vi "编辑输出控件.vi"(8 "error in (no error)":errorcluster caption="错误输入（无错误）", 11 "程序响应 输入":refnum<class "程序响应.lvclass">) -> (0 "error out":errorcluster caption="错误输出", 3 "程序响应 输出":refnum<class "程序响应.lvclass">)   [LabVIEW 2016]
uses:
  C:/Program Files (x86)/National Instruments/LabVIEW 2016/vi.lib/ActorFramework/Actor/Actor.lvclass
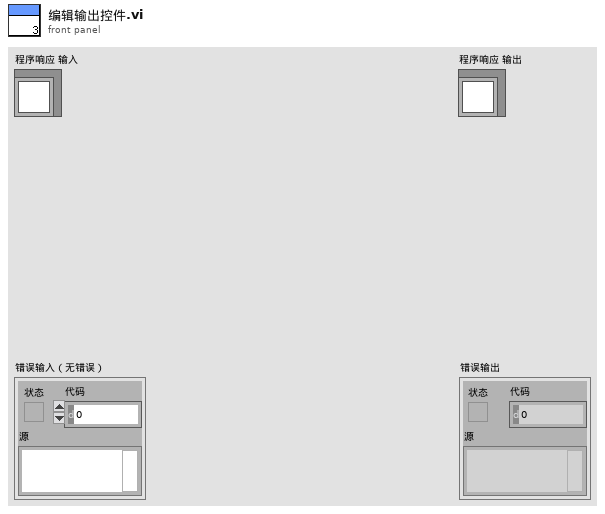
[diagram p1: front panel]
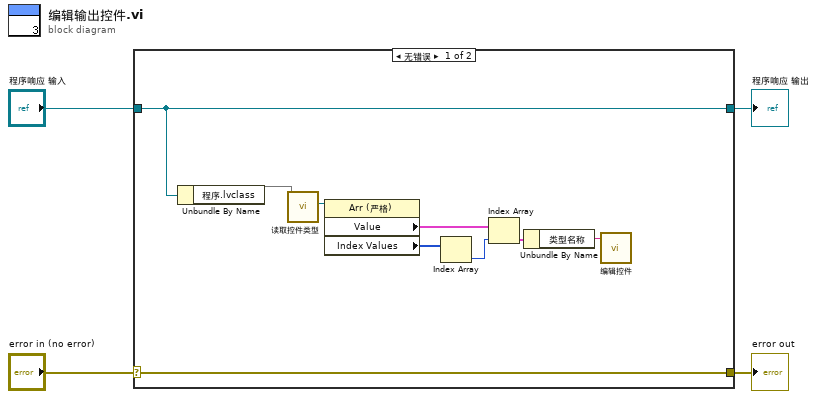
[diagram p0: block diagram]
diagram:
  n1 = case shown="无错误" "error in (no error)" {
    selector: "error in (no error)" -> [w13 w15]
    tunnel: [w13 w15] -> w3
    tunnel: [w12 w14] -> w1
    tunnel: "程序响应 输入" -> [w12 w14]
    frame No Error {
      n2 = Unbundle By Name(w12) -> ("程序.lvclass"=w11)
      n3 = call-dynamic "读取控件类型.vi"("程序输入"=w11) -> ("控件类型"=w10:refnum<vi>)  [unwired: 8 in, 2 out]
      n4 = property class="Arr (严格)"(reference=w10) -> ("Value"=w8:cluster{"二维图片":picture, "类型名称":string}[], "Index Values"=w9:u32[])  [unwired: 1 in, 2 out]
      n5 = Index Array(array=w9) -> (element=w7:u32)  [unwired: 1 in]
      n6 = Index Array(array=w8, index=w7) -> (element=w6:cluster{"二维图片":picture, "类型名称":string})
      n7 = Unbundle By Name(w6) -> ("类型名称"=w5:string)
      n8 = call "编辑控件.vi"("控件类型"=w5) -> ()  [unwired: 11 in]
    }
    frame Error {
    }
  }
  "error out" <- w3
  "程序响应 输出" <- w1
